vi "FormulaNodeSample.vi"() -> ()   [LabVIEW 2025]
doc: "Uses a Formula Node within a subVI to perform complex mathematical operations, allowing reusable calculation logic."
panel:
  in  "c":dbl
  in  "b":dbl
  out "f":dbl
  in  "a":dbl
  in  "x":dbl
  # "Using formula node implemented complex mathematical operation using subvi"
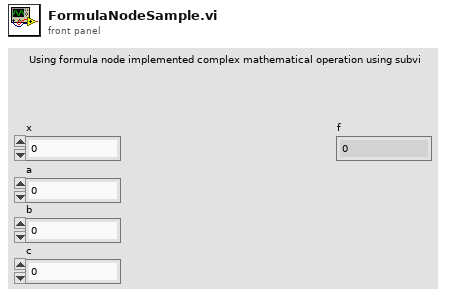
[diagram p1: front panel]
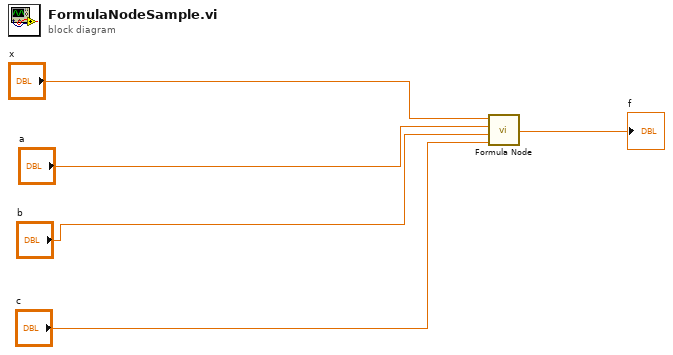
[diagram p0: block diagram]
diagram:
  n1 = call "Formula Node.vi"("c"="c", "b"="b", "a"="a", "x"="x") -> ("f"=→"f":dbl)
